vi "Read Accelerometer Values And Light LED And Write to Serial.vi"() -> ()   [LabVIEW 2014]
doc: "Tested on:\n - Arduino Nano\n - WemosD1 with ESP8266\n\nSending raw accelerometer data through UART to computer."
uses:
  <vilib>/LabVIEW Universal Transcriptor/LabVIEW to Arduino Transcriptor/Transcriptors/System API/Serial println string.vi
  <vilib>/LabVIEW Universal Transcriptor/Arduino MPU6050 Library/Arduino MPU6050.lvlib
panel:
  in  "serial speed (Bd)":i32=115200
  in  "address":u16(ring)=104 items=["AD0 pin NOT CONNECTED"=104, "AD0 connect to Vcc"=105]
  in  "range":T1(ring)
  in  "scale":T2(ring)
  in  "Error In":errorcluster
  out "error out":errorcluster
  # "Wiring:\nMPU6050 | WemosD1 | Arduino\n        |         | Nano\n--------+---------+----------\nVcc     | +5V     | +5V\nGND     | GND     | GND\nSCL     | D15/SCL | A5\nSDA     | D14/SCA | A4\nSCA     | D14/SDA"
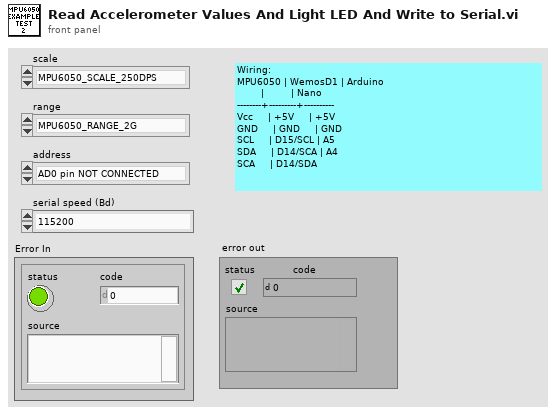
[diagram p1: front panel]
types:
  T1 = enum16{"MPU6050_RANGE_2G", "MPU6050_RANGE_4G", "MPU6050_RANGE_8G", "MPU6050_RANGE_16G"}
  T2 = enum16{"MPU6050_SCALE_250DPS", "MPU6050_SCALE_500DPS", "MPU6050_SCALE_1000DPS", "MPU6050_SCALE_2000DPS"}
  T3 = typedef "Arduino MPU6050.lvlib/MPU6050LibVector.ctl" = cluster{"XAxis":sgl, "YAxis":sgl, "ZAxis":sgl}
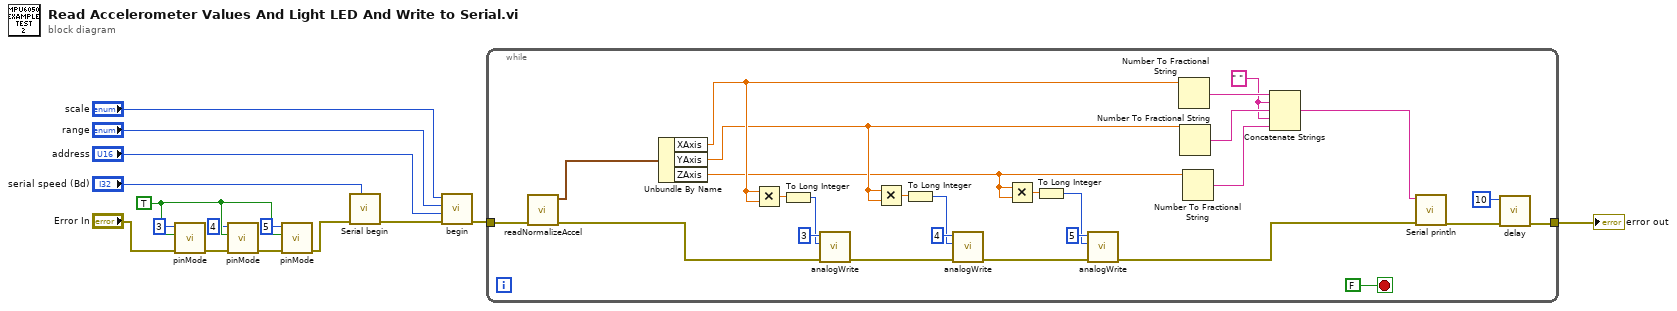
[diagram p0: block diagram]
diagram:
  w4 = TRUE ("output?")
  n1 = call <vilib>:"pinMode.vi"("Error In"="Error In", "output?"=w4, "pin number"=3) -> ("Error Out"=w6:errorcluster)  [unwired: 8 in]
  n2 = call <vilib>:"pinMode.vi"("Error In"=w6, "output?"=w4, "pin number"=4) -> ("Error Out"=w8:errorcluster)  [unwired: 8 in]
  n3 = call <vilib>:"pinMode.vi"("Error In"=w8, "output?"=w4, "pin number"=5) -> ("Error Out"=w5:errorcluster)  [unwired: 8 in]
  n4 = call <vilib>:"Serial begin.vi"("Error In"=w5, "speed (Bd)"="serial speed (Bd)") -> ("Error Out"=w14:errorcluster)  [unwired: 9 in]
  n5 = call <vilib>:"begin.vi"("Error In"=w14, "address"="address", "range"="range", "scale"="scale") -> ("Error Out"=w9:errorcluster)  [unwired: 7 in]
  n6 = while {
    tunnel: w9 -> [w33]
    tunnel: [w41] -> w15
    stop <- FALSE stop-if-true
    w34 = " " ("F-format string")
    n7 = call <vilib>:"readNormalizeAccel.vi"("error in (no error)"=w33) -> ("error out"=w29:errorcluster, "Vector"=w32:T3)  [unwired: 9 in]
    n8 = Unbundle By Name(w32) -> ("XAxis"=w24:sgl, "YAxis"=w19:sgl, "ZAxis"=w16:sgl)
    n9 = Multiply(x=w24, y=w24) -> (x*y=w23:sgl)
    n10 = To Long Integer(number=w23) -> (32bit integer=w22:i32)
    n11 = call <vilib>:"analogWrite.vi"("Error In"=w29, "value"=w22, "pin number"=3) -> ("Error Out"=w31:errorcluster)  [unwired: 8 in]
    n12 = Multiply(x=w19, y=w19) -> (x*y=w21:sgl)
    n13 = To Long Integer(number=w21) -> (32bit integer=w20:i32)
    n14 = call <vilib>:"analogWrite.vi"("Error In"=w31, "value"=w20, "pin number"=4) -> ("Error Out"=w30:errorcluster)  [unwired: 8 in]
    n15 = Multiply(x=w16, y=w16) -> (x*y=w18:sgl)
    n16 = To Long Integer(number=w18) -> (32bit integer=w17:i32)
    n17 = call <vilib>:"analogWrite.vi"("Error In"=w30, "value"=w17, "pin number"=5) -> ("Error Out"=w28:errorcluster)  [unwired: 8 in]
    n18 = Number To Fractional String(number=w24) -> (F-format string=w38:string)  [unwired: 3 in]
    n19 = Number To Fractional String(number=w19) -> (F-format string=w37:string)  [unwired: 3 in]
    n20 = Number To Fractional String(number=w16) -> (F-format string=w36:string)  [unwired: 3 in]
    n21 = Concatenate Strings(w38, w34, w37, w34, w36) -> (w35:string)
    n22 = call-poly <vilib>:"Serial println.vi"("Error In"=w28, "string in"=w35) -> ("Error Out"=w40:errorcluster)  [unwired: 9 in]
    n23 = call <vilib>:"delay.vi"("Error In"=w40, "time (ms)"=10) -> ("Error Out"=w41:errorcluster)  [unwired: 9 in]
  }
  "error out" <- w15
